vi "DPO_7K_Set_Sampling_Mode.vi"(8 "Error In":errorcluster, 10 "Sampling Mode":u16(ring) items=["Real Time", "Equivalent Time", "Interpolation"], 11 "VISA resource name in":refnum<visa-resource-name>) -> (0 "Error Out":errorcluster, 3 "VISA resource name out":refnum<visa-resource-name>)   [LabVIEW 2020]
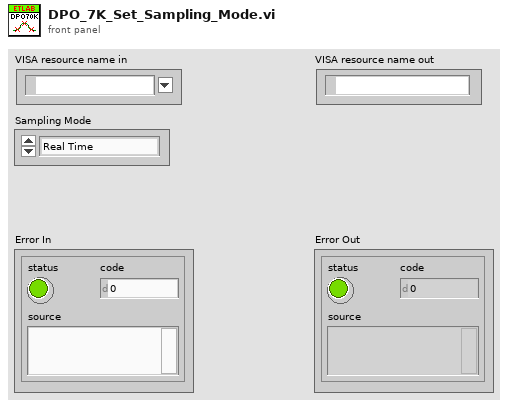
[diagram p1: front panel]
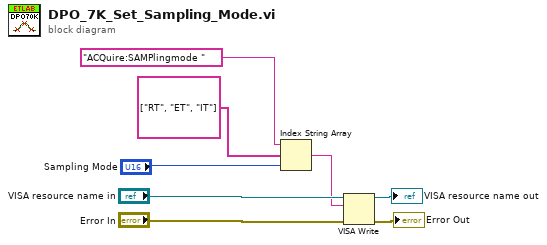
[diagram p0: block diagram]
diagram:
  n1 = Index String Array(1:"Sampling Mode", 2:string[] ["RT", "ET", "IT"], 3:"ACQuire:SAMPlingmode ") -> (0:w2:string)
  n2 = VISA Write(VISA resource name="VISA resource name in", write buffer=w2, error in (no error)="Error In") -> (VISA resource name out=→"VISA resource name out":refnum<visa-resource-name>, error out=→"Error Out":errorcluster)  [unwired: 1 out]
